vi "Update_Matlab_for_calib.vi"(8 "error in (no error)":errorcluster, 11 "Current Calibration Parameters":T1) -> (0 "error out":errorcluster)   [LabVIEW 2020]
uses:
  TypeDefs/Current Calibration Parameters.ctl
  Global Variables/General Globals.vi
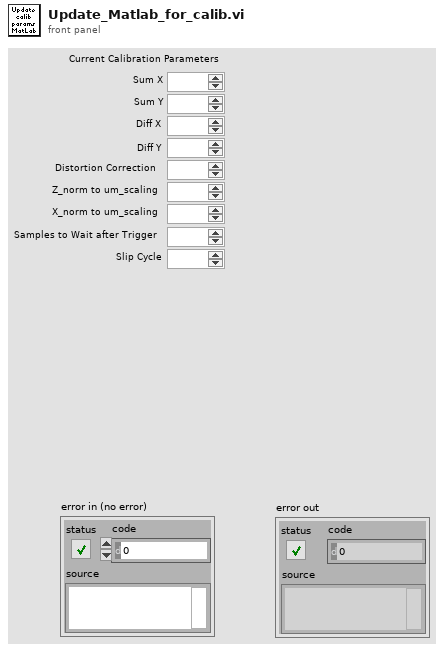
[diagram p1: front panel]
types:
  T1 = typedef "Current Calibration Parameters.ctl" = cluster{"Sum X":dbl, "Sum Y":dbl, "Diff X":dbl, "Diff Y":dbl, "Distortion Correction":dbl, "Z_norm to um_scaling":dbl, "X_norm to um_scaling":dbl, "Samples to Wait after Trigger":dbl, "Slip Cycle":dbl}
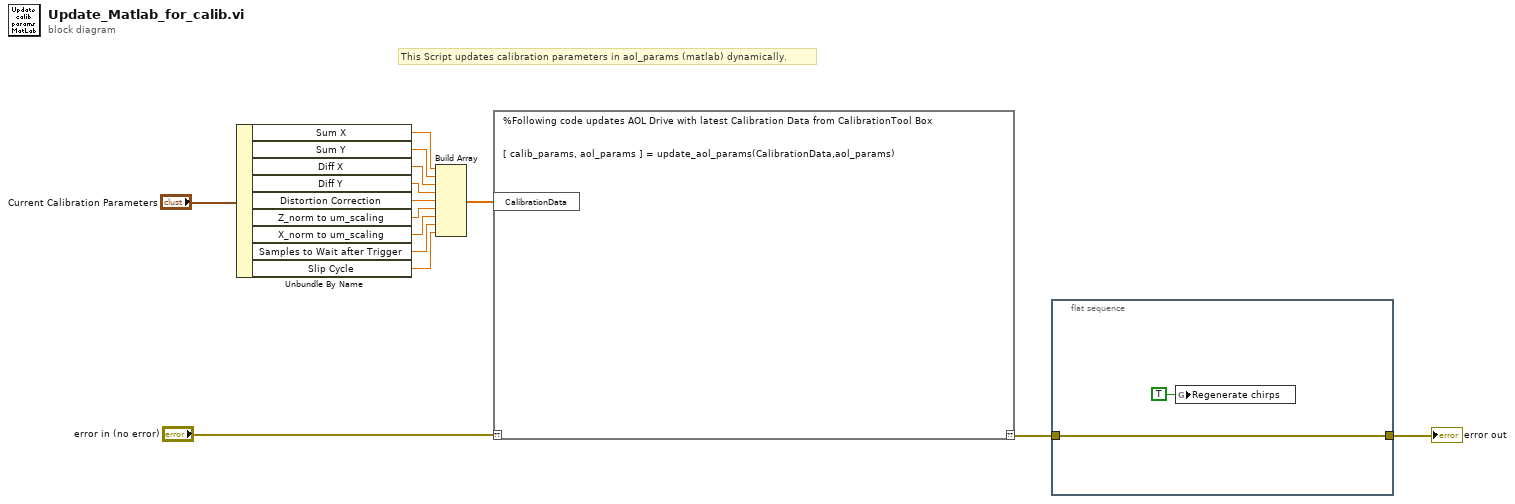
[diagram p0: block diagram]
diagram:
  # "This Script updates calibration parameters in aol_params (matlab) dynamically."
  n1 = Unbundle By Name("Current Calibration Parameters") -> ("Sum X"=w12:dbl, "Sum Y"=w11:dbl, "Diff X"=w10:dbl, "Diff Y"=w9:dbl, "Distortion Correction"=w8:dbl, "Z_norm to um_scaling"=w7:dbl, "X_norm to um_scaling"=w6:dbl, "Samples to Wait after Trigger"=w5:dbl, "Slip Cycle"=w4:dbl)
  n2 = Build Array(w12, w11, w10, w9, w8, w7, w6, w5, w4) -> (w3:dbl[])
  n3 = script code="%Following code updates AOL Drive with latest Calibration Data from CalibrationTool Box\n\n\n[ calib_params, aol_params ] = update_aol_params(CalibrationData,aol_params)"("??"="error in (no error)", "CalibrationData"=w3) -> ("??"=w2:errorcluster)
  n4 = flat-sequence {
    tunnel: w2 -> [w16]
    tunnel: [w16] -> w1
    frame #0 {
      n5 = global write "General Globals.vi" "Regenerate chirps"(TRUE ("Regenerate chirps")) -> ()
    }
  }
  "error out" <- w1
